vi "Save_Data.vi"(0 "保存路径":path=path "C:/Qmz/data1.bin", 3 "Save Data":bool) -> ()   [LabVIEW 2020]
uses:
  <vilib>/Platform/TimedLoop/XDataNode/timing_clust.ctl
  <vilib>/Platform/TimedLoop/XDataNode/nitl_modes.ctl
  <vilib>/Platform/TimedLoop/XDataNode/wakeup.ctl
  <vilib>/Platform/TimedLoop/XDataNode/XDataNode.xnode
  <vilib>/Platform/TimedLoop/XDataNode/XDNodeRunTimeDep.lvlib
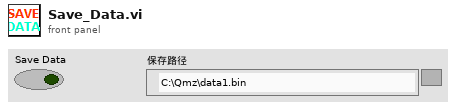
[diagram p1: front panel]
types:
  T1 = enum16{"open", "replace", "create", "open or create", "replace or create", "replace or create with confirmation"}
  T2 = typedef "XDNodeRunTimeDep.lvlib/timing_clust.ctl" = cluster{"Expected End [f-1]":u64, "Actual End [f-1]":u64, "Finished Late? [f-1]":bool, "Expected End [i-1]":u64, "Actual End [i-1]":u64, "Finished Late? [i-1]":bool, "Expected Start [i]":u64, "Actual Start [i]":u64, "Expected Start [f]":u64, "Actual Start [f]":u64, "Source Name":string, "Structure Name":string, "Period":i64, "Deadline":i64, "Offset":i64, "Start":i64, "Priority":i32, "Timeout":i32, "Mode":T3, "Wakeup Reason":T4, "Error":errorcluster, "Source Type":string, "Secondary Source Type":string, "Global End Time":u64, "Global Start Time":u64, "Frame Duration":u64, "Iteration Duration":u64, "Assigned CPU":i32, "I/O Scan Engine Mode":u32}
  T3 = typedef "XDNodeRunTimeDep.lvlib/nitl_modes.ctl" = enum32{"No Change", "Process missed periods, maintain original phase", "Discard missed periods, maintain original phase", "Process missed periods, ignore original phase", "Discard missed periods, ignore original phase"}
  T4 = typedef "XDNodeRunTimeDep.lvlib/wakeup.ctl" = enum32{"Normal", "Aborted", "Asynchronous wakeup", "Timing source error", "Timed loop error", "Timeout"}
  T5 = enum16{"big-endian, network order", "native, host order", "little-endian"}
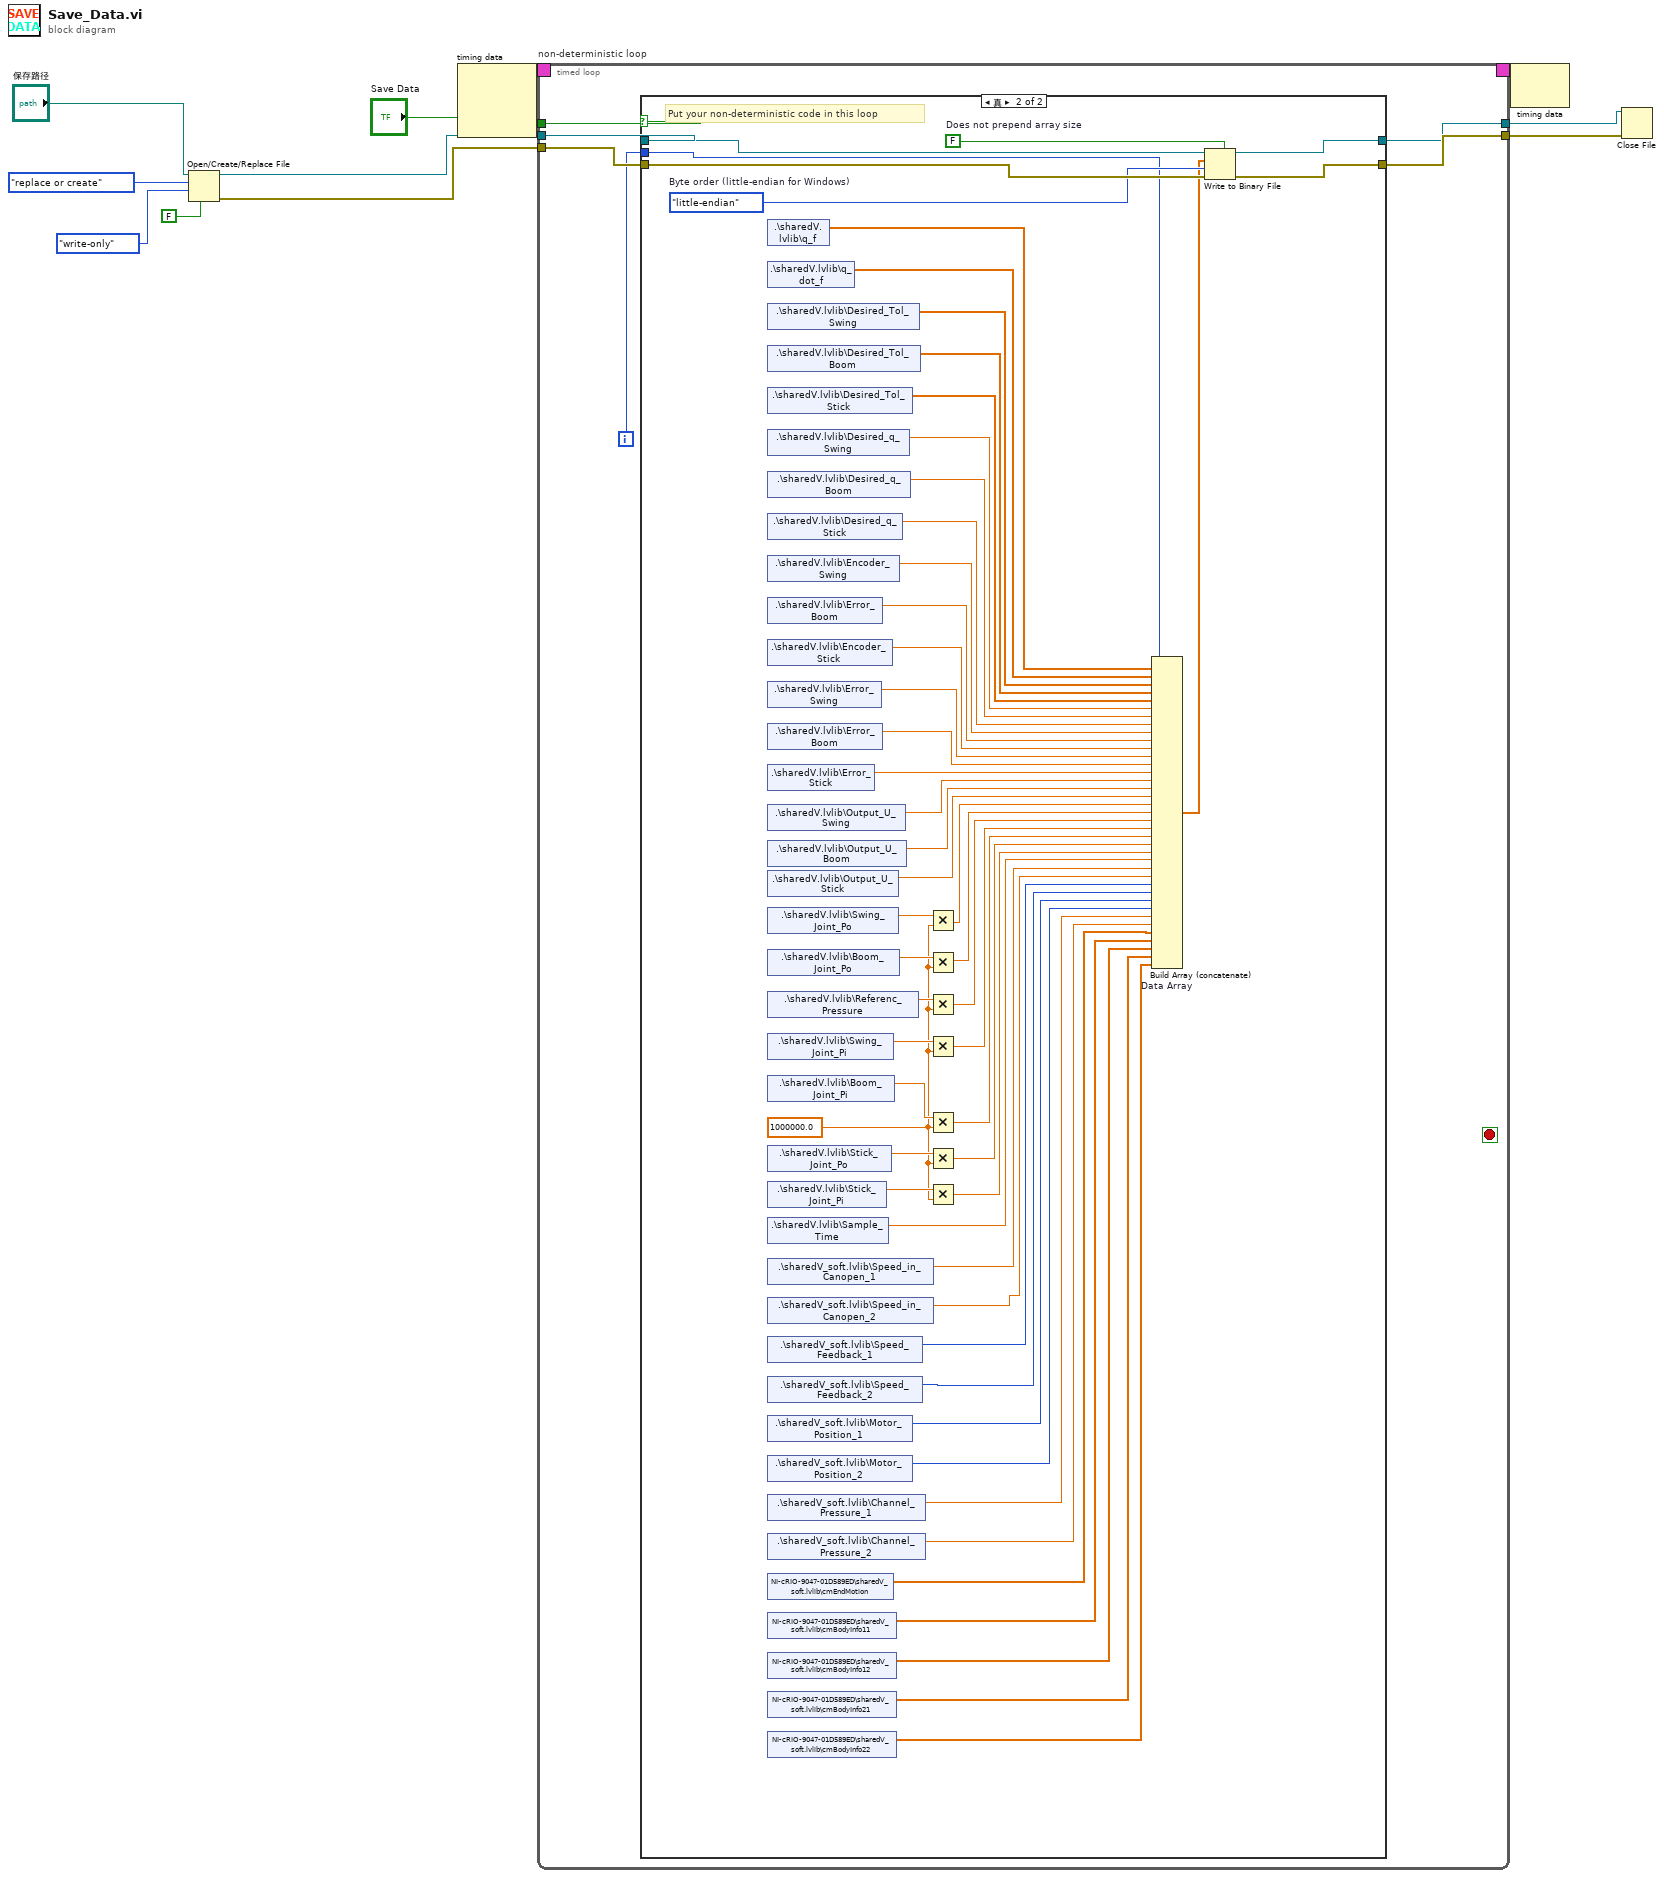
[diagram p0: block diagram]
diagram:
  n1 = Open/Create/Replace File(file path (use dialog)="保存路径", operation (0:open)=T1."replace or create", access (0:read/write)=enum16{"read/write", "read-only", "write-only"}."write-only" ("权限(0:read/write)"), disable buffering (F)=FALSE) -> (refnum out=w7:refnum<file>, error out=w6:errorcluster)  [unwired: 2 in, 1 out]
  n2 = node-c288 ("Input Node")() -> (w11:T2)  [unwired: 3 in]
  n3 = timed-loop "non-deterministic loop" {
    timing: w11 -> [_]
    timing-out: [_] -> w10
    tunnel: [w17] -> w4
    tunnel: w6 -> [w16]
    tunnel: [w15] -> w5
    tunnel: "Save Data" -> [w14]
    tunnel: w7 -> [w13]
    i -> [w12]
    stop <- _ stop-if-true
    n4 = case shown="真" w14 {
      tunnel: [w18 w73] -> w17
      tunnel: w13 -> [w19 w72]
      tunnel: w16 -> [w18 w71]
      tunnel: [w19 w68] -> w15
      tunnel: w12 -> [_ w66]
      frame False {
      }
      frame True {
        w44 = 1000000.0
        w69 = FALSE  # Does not prepend array size
        w70 = T5."little-endian"  # Byte order (little-endian for Windows)
        # "Put your non-deterministic code in this loop"
        n5 = shared-variable ".\\sharedV.lvlib\\q_f"() -> (w65:dbl[])  [unwired: 1 in, 1 out]
        n6 = shared-variable ".\\sharedV.lvlib\\q_dot_f"() -> (w64:dbl[])  [unwired: 1 in, 1 out]
        n7 = shared-variable ".\\sharedV.lvlib\\Desired_Tol_Swing"() -> (w63:dbl[])  [unwired: 1 in, 1 out]
        n8 = shared-variable ".\\sharedV.lvlib\\Desired_Tol_Boom"() -> (w62:dbl[])  [unwired: 1 in, 1 out]
        n9 = shared-variable ".\\sharedV.lvlib\\Desired_Tol_Stick"() -> (w61:dbl[])  [unwired: 1 in, 1 out]
        n10 = shared-variable ".\\sharedV.lvlib\\Desired_q_Swing"() -> (w60:dbl)  [unwired: 1 in, 1 out]
        n11 = shared-variable ".\\sharedV.lvlib\\Desired_q_Boom"() -> (w59:dbl)  [unwired: 1 in, 1 out]
        n12 = shared-variable ".\\sharedV.lvlib\\Desired_q_Stick"() -> (w58:dbl)  [unwired: 1 in, 1 out]
        n13 = shared-variable ".\\sharedV.lvlib\\Encoder_Swing"() -> (w57:dbl)  [unwired: 1 in, 1 out]
        n14 = shared-variable ".\\sharedV.lvlib\\Error_Boom"() -> (w56:dbl)  [unwired: 1 in, 1 out]
        n15 = shared-variable ".\\sharedV.lvlib\\Encoder_Stick"() -> (w55:dbl)  [unwired: 1 in, 1 out]
        n16 = shared-variable ".\\sharedV.lvlib\\Error_Swing"() -> (w54:dbl)  [unwired: 1 in, 1 out]
        n17 = shared-variable ".\\sharedV.lvlib\\Error_Boom"() -> (w53:dbl)  [unwired: 1 in, 1 out]
        n18 = shared-variable ".\\sharedV.lvlib\\Error_Stick"() -> (w52:dbl)  [unwired: 1 in, 1 out]
        n19 = shared-variable ".\\sharedV.lvlib\\Output_U_Swing"() -> (w43:dbl)  [unwired: 1 in, 1 out]
        n20 = shared-variable ".\\sharedV.lvlib\\Output_U_Boom"() -> (w42:dbl)  [unwired: 1 in, 1 out]
        n21 = shared-variable ".\\sharedV.lvlib\\Output_U_Stick"() -> (w41:dbl)  [unwired: 1 in, 1 out]
        n22 = shared-variable ".\\sharedV.lvlib\\Swing_Joint_Po"() -> (w51:dbl)  [unwired: 1 in, 1 out]
        n23 = shared-variable ".\\sharedV.lvlib\\Boom_Joint_Po"() -> (w49:dbl)  [unwired: 1 in, 1 out]
        n24 = shared-variable ".\\sharedV.lvlib\\Referenc_Pressure"() -> (w45:dbl)  [unwired: 1 in, 1 out]
        n25 = shared-variable ".\\sharedV.lvlib\\Swing_Joint_Pi"() -> (w50:dbl)  [unwired: 1 in, 1 out]
        n26 = shared-variable ".\\sharedV.lvlib\\Boom_Joint_Pi"() -> (w48:dbl)  [unwired: 1 in, 1 out]
        n27 = shared-variable ".\\sharedV.lvlib\\Stick_Joint_Po"() -> (w47:dbl)  [unwired: 1 in, 1 out]
        n28 = shared-variable ".\\sharedV.lvlib\\Stick_Joint_Pi"() -> (w46:dbl)  [unwired: 1 in, 1 out]
        n29 = shared-variable ".\\sharedV.lvlib\\Sample_Time"() -> (w33:dbl)  [unwired: 1 in, 1 out]
        n30 = shared-variable ".\\sharedV_soft.lvlib\\Speed_in_Canopen_1"() -> (w32:dbl)  [unwired: 1 in, 1 out]
        n31 = shared-variable ".\\sharedV_soft.lvlib\\Speed_in_Canopen_2"() -> (w31:dbl)  [unwired: 1 in, 1 out]
        n32 = shared-variable ".\\sharedV_soft.lvlib\\Speed_Feedback_1"() -> (w30:i32)  [unwired: 1 in, 1 out]
        n33 = shared-variable ".\\sharedV_soft.lvlib\\Speed_Feedback_2"() -> (w29:i32)  [unwired: 1 in, 1 out]
        n34 = shared-variable ".\\sharedV_soft.lvlib\\Motor_Position_1"() -> (w28:i32)  [unwired: 1 in, 1 out]
        n35 = shared-variable ".\\sharedV_soft.lvlib\\Motor_Position_2"() -> (w27:i32)  [unwired: 1 in, 1 out]
        n36 = shared-variable ".\\sharedV_soft.lvlib\\Channel_Pressure_1"() -> (w26:dbl)  [unwired: 1 in, 1 out]
        n37 = shared-variable ".\\sharedV_soft.lvlib\\Channel_Pressure_2"() -> (w25:dbl)  [unwired: 1 in, 1 out]
        n38 = shared-variable "NI-cRIO-9047-01D589ED\\sharedV_soft.lvlib\\cmEndMotion"() -> (w24:dbl[])  [unwired: 1 in, 1 out]
        n39 = shared-variable "NI-cRIO-9047-01D589ED\\sharedV_soft.lvlib\\cmBodyInfo11"() -> (w23:dbl[])  [unwired: 1 in, 1 out]
        n40 = shared-variable "NI-cRIO-9047-01D589ED\\sharedV_soft.lvlib\\cmBodyInfo12"() -> (w22:dbl[])  [unwired: 1 in, 1 out]
        n41 = shared-variable "NI-cRIO-9047-01D589ED\\sharedV_soft.lvlib\\cmBodyInfo21"() -> (w21:dbl[])  [unwired: 1 in, 1 out]
        n42 = shared-variable "NI-cRIO-9047-01D589ED\\sharedV_soft.lvlib\\cmBodyInfo22"() -> (w20:dbl[])  [unwired: 1 in, 1 out]
        n43 = Multiply(x=w51, y=w44) -> (x*y=w40:dbl)
        n44 = Multiply(x=w49, y=w44) -> (x*y=w39:dbl)
        n45 = Multiply(x=w45, y=w44) -> (x*y=w38:dbl)
        n46 = Multiply(x=w50, y=w44) -> (x*y=w37:dbl)
        n47 = Multiply(x=w48, y=w44) -> (x*y=w36:dbl)
        n48 = Multiply(x=w47, y=w44) -> (x*y=w35:dbl)
        n49 = Multiply(x=w46, y=w44) -> (x*y=w34:dbl)
        n50 = Build Array (concatenate) "Data Array"(w66, w65, w64, w63, w62, w61, w60, w59, w58, w57, w56, w55, w54, w53, w52, w43, w42, w41, w40, w39, w38, w37, w36, w35, w34, w33, w32, w31, w30, w29, w28, w27, w26, w25, w24, w23, w22, w21, w20) -> (w67:dbl[])
        n51 = Write to Binary File(file (use dialog)=w72, data=w67, error in=w71, 5:w69, 9:w70) -> (refnum out=w68:refnum<file>, error out=w73:errorcluster)  [unwired: 1 in, 1 out]
      }
    }
  }
  n52 = node-c288 ("Output Node")(w10) -> ()  [unwired: 1 out]
  n53 = Close File(refnum=w5, error in=w4) -> ()  [unwired: 2 out]
